vi "模拟输入_连续(换算).vi"() -> ()   [LabVIEW 2013]
doc: "This example demonstrates how to acquire a continuous data."
uses:
  <userlib>/ArtDAQ/_SubVI/ArtDAQ_CreateAIVoltageChan.vi
  <userlib>/ArtDAQ/_SubVI/ArtDAQ_CfgSampClkTiming.vi
  <userlib>/ArtDAQ/_SubVI/ArtDAQ_Read Analog DBL NChan NSamp.vi
panel:
  out "错误输出":errorcluster
  in  "停止":bool
  out "Waveform":dbl[][](graph)
  in  "采样频率":dbl=10000.0 format="%#_13g"
  in  "每通道采样点数":i32=1000
  in  "接地方式":i32(ring)=10083 items=["默认"=-1, "单端"=10083, "非参考单端"=10078, "差分"=10106, "伪差分"=12529]
  in  "最小值(V)":dbl=-10.0 format="%#_13g"
  in  "最大值(V)":dbl=10.0 format="%#_13g"
  in  "物理通道":string(combo)="Dev1/ai0"
  # "通道属性"
  # "定时"
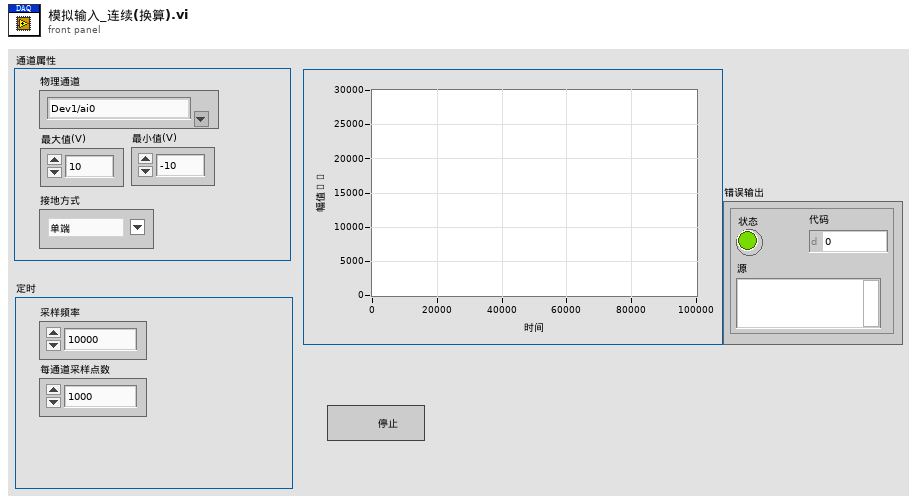
[diagram p1: front panel]
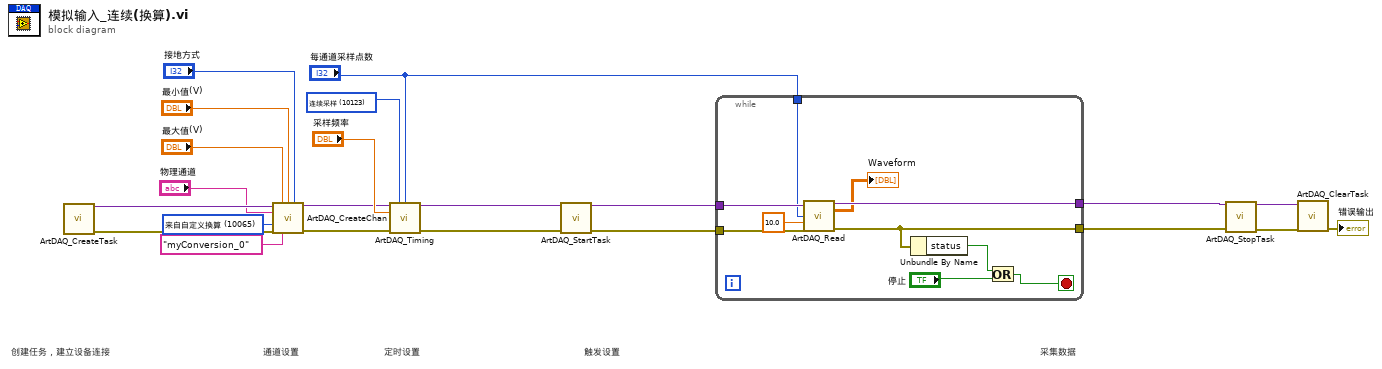
[diagram p0: block diagram]
diagram:
  w4 = 10065 items=["V"=10348, "来自自定义换算"=10065] ("单位")
  w10 = 10123 items=["有限点采样"=10178, "连续采样"=10123] ("SampleMode")
  # "采集数据"
  # "触发设置"
  # "定时设置"
  # "通道设置"
  # "创建任务，建立设备连接"
  n1 = call <userlib>:"ArtDAQ_CreateTask.vi"() -> ("任务句柄"=w15:variant, "错误输出"=w22:errorcluster)  [unwired: 14 in]
  n2 = call-poly <userlib>:"ArtDAQ_CreateChan.vi"("任务句柄"=w15, "最大值"="最大值(V)", "最小值"="最小值(V)", "接线端配置"="接地方式", "物理通道"="物理通道", "单位"=w4, "错误输入"=w22, "自定义换算名称"="myConversion_0") -> ("任务句柄"=w11:variant, "错误输出"=w18:errorcluster)  [unwired: 6 in]
  n3 = call-poly <userlib>:"ArtDAQ_Timing.vi"("任务句柄"=w11, "采样模式"=w10, "每通道采样数"="每通道采样点数", "采样率"="采样频率", "错误输入"=w18) -> ("任务句柄"=w9:variant, "错误输出"=w8:errorcluster)  [unwired: 9 in]
  n4 = call <userlib>:"ArtDAQ_StartTask.vi"("任务句柄"=w9, "错误输入"=w8) -> ("任务句柄"=w2:variant, "错误输出"=w16:errorcluster)  [unwired: 12 in]
  n5 = while {
    tunnel: w2 -> [w32]
    tunnel: w16 -> [w31]
    tunnel: "每通道采样点数" -> [w30]
    tunnel: [w28] -> w1
    tunnel: [w27] -> w14
    stop <- w23 stop-if-true
    n6 = call-poly <userlib>:"ArtDAQ_Read.vi"("任务句柄"=w32, "每通道采样数"=w30, "超时s"=10.0 ("Timeout"), "错误输入"=w31) -> ("任务句柄"=w28:variant, "数据"=→"Waveform":dbl[][], "错误输出"=w27:errorcluster)  [unwired: 8 in, 1 out]
    n7 = Unbundle By Name(w27) -> ("status"=w26:bool)
    n8 = Or(x=w26, y="停止") -> (x .or. y?=w23:bool)
  }
  n9 = call <userlib>:"ArtDAQ_StopTask.vi"("任务句柄"=w1, "错误输入"=w14) -> ("任务句柄"=w13:variant, "错误输出"=w12:errorcluster)  [unwired: 12 in]
  n10 = call <userlib>:"ArtDAQ_ClearTask.vi"("任务句柄"=w13, "错误输入"=w12) -> ("错误输出"=→"错误输出":errorcluster)  [unwired: 13 in]
